vi "Set Setpoint Paramters.vi"(7 "setpoint":string, 8 "error in (no error)":errorcluster, 11 "setpoint cluster":T1={"open-loop controls"={"high pw"=5.0, "low pw"=5.8}, "ramp controls"={"systole"=0.8, "diastole"=0.2}, "blood-pressure controls"={"systole"=0.8, "systole 2"=0.2, "systole 3"=1.0, "systole 4"=0.6}, "sinusoidal controls"={"systole"=0.0, "systole 2"=0.0, "systole 3"=0.0}}) -> (0 "error out":errorcluster, 3 "IA test param out":refnum<class "IA Test Parameters.lvclass">)   [LabVIEW 2020]
uses:
  Parameter Class/IA Test Parameters.lvclass
  Parameter Class/Setpoints/Setpoint Cluster.ctl
  Controls/Open Loop Controls.ctl
  Controls/Ramp Controls.ctl
  Controls/Blood Pressure Controls.ctl
  Controls/sinusoidal controls.ctl
  Parameter Class/Setpoints/Open-loop/Open-Loop Setpoint.lvclass
  C:/Users/jharw/Documents/1 Folder to Rule them All/UMD/Inflation-Apparatus/src/Inflation Test/Parameter Class/IA Test Parameters.lvclass
  Parameter Class/Setpoints/Open-loop/Open-Loop Setpoint.lvclass/Open-Loop Setpoint.ctl
  Parameter Class/Setpoints/Ramp Setpoint/Ramp Setpoint.lvclass
  Parameter Class/Setpoints/Ramp Setpoint/Ramp Setpoint.lvclass/Ramp Setpoint.ctl
  C:/Users/jharw/Documents/1 Folder to Rule them All/UMD/Inflation-Apparatus/src/Inflation Test/Parameter Class/Setpoints/Open-loop/Open-Loop Setpoint.lvclass
  C:/Users/jharw/Documents/1 Folder to Rule them All/UMD/Inflation-Apparatus/src/Inflation Test/Parameter Class/Setpoints/Ramp Setpoint/Ramp Setpoint.lvclass
panel:
  # "SYSTOLE (V):"
  # "DIASTOLE (V):"
  # "FREQUENCY (HZ):"
  # "SYSTOLE (V):"
  # "DIASTOLE (V):"
  # "DICROTIC NOTCH (V):"
  # "FREQUENCY (HZ):"
  # "SYSTOLE (V):"
  # "DIASTOLE (V):"
  # "HIGH PW (%):"
  # "LOW PW (%):"
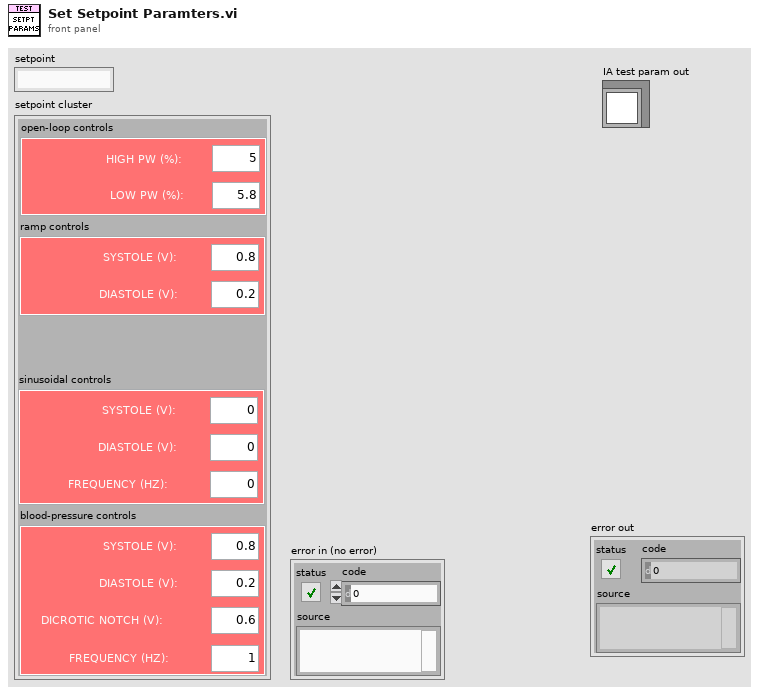
[diagram p1: front panel]
types:
  T1 = typedef "Setpoint Cluster.ctl" = cluster{"open-loop controls":T2, "ramp controls":T3, "blood-pressure controls":T4, "sinusoidal controls":T5}
  T2 = typedef "Open Loop Controls.ctl" = cluster{"high pw":dbl, "low pw":dbl}
  T3 = typedef "Ramp Controls.ctl" = cluster{"systole":dbl, "diastole":dbl}
  T4 = typedef "Blood Pressure Controls.ctl" = cluster{"systole":dbl, "systole 2":dbl, "systole 3":dbl, "systole 4":dbl}
  T5 = typedef "sinusoidal controls.ctl" = cluster{"systole":dbl, "systole 2":dbl, "systole 3":dbl}
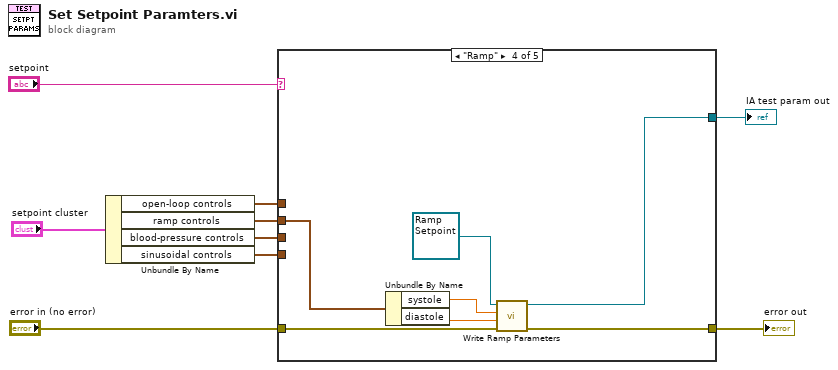
[diagram p0: block diagram]
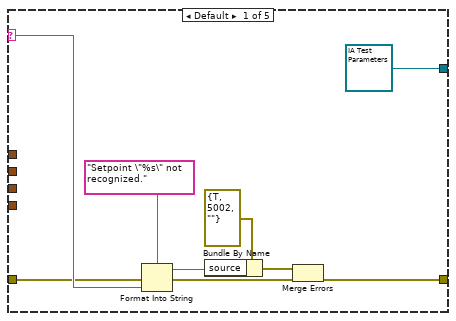
[diagram p2: hidden frame]
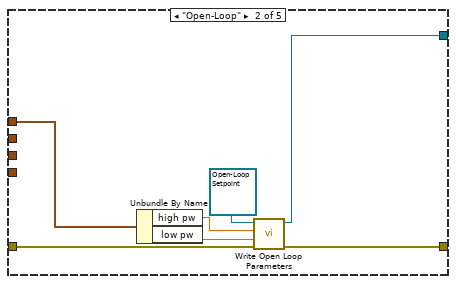
[diagram p3: hidden frame]
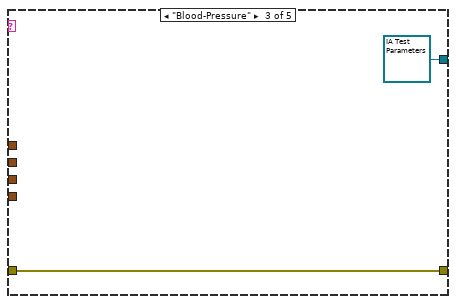
[diagram p4: hidden frame]
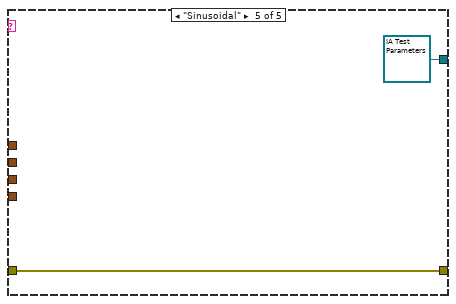
[diagram p5: hidden frame]
diagram:
  n1 = Unbundle By Name("setpoint cluster") -> ("open-loop controls"=w4:T2, "ramp controls"=w3:T3, "blood-pressure controls"=w2:T4, "sinusoidal controls"=w1:T5)
  n2 = case shown="\"Ramp\"" "setpoint" {
    selector: "setpoint" -> [w13 _ _ _ _]
    tunnel: [refnum<class "IA Test Parameters.lvclass"> refnum ("IA Test Parameters.lvclass") w22 refnum<class "IA Test Parameters.lvclass"> refnum ("IA Test Parameters.lvclass") w29 refnum<class "IA Test Parameters.lvclass"> refnum ("IA Test Parameters.lvclass")] -> w6
    tunnel: "error in (no error)" -> [w11 w25 w27 w33 w35]
    tunnel: [w12 w24 w27 w32 w35] -> w9
    tunnel: w4 -> [_ w19 _ _ _]
    tunnel: w3 -> [_ _ _ w28 _]
    tunnel: w2 -> [_ _ _ _ _]
    tunnel: w1 -> [_ _ _ _ _]
    frame Default {
      n3 = Format Into String(format string="Setpoint \"%s\" not recognized.", error in=w11, w13) -> (resulting string=w17:string, error out=w15:errorcluster)  [unwired: 1 in]
      n4 = Bundle By Name(cluster=errorcluster {"status"=TRUE, "code"=5002, "source"=""} ("error out"), "source"=w17) -> (w14:errorcluster)
      n5 = Merge Errors(w14, w15) -> (w12:errorcluster)
    }
    frame "Open-Loop" {
      n6 = Unbundle By Name(w19) -> ("high pw"=w20:dbl, "low pw"=w21:dbl)
      n7 = call "Write Open Loop Parameters.vi"("error in (no error)"=w25, "Low PW"=w21, "High-PW"=w20, "Open-Loop Setpoint in"=refnum<class "Open-Loop Setpoint.lvclass"> refnum) -> ("error out"=w24:errorcluster, "Open-Loop Setpoint out"=w22:refnum<class "Open-Loop Setpoint.lvclass">)  [unwired: 6 in]
    }
    frame "Blood-Pressure" {
    }
    frame "Ramp" {
      n8 = Unbundle By Name(w28) -> ("systole"=w30:dbl, "diastole"=w31:dbl)
      n9 = call "Write Ramp Parameters.vi"("error in (no error)"=w33, "diastole"=w31, "systole"=w30, "Ramp Setpoint in"=refnum<class "Ramp Setpoint.lvclass"> refnum ("Ramp Setpoint.lvclass")) -> ("error out"=w32:errorcluster, "Ramp Setpoint out"=w29:refnum<class "Ramp Setpoint.lvclass">)  [unwired: 6 in]
    }
    frame "Sinusoidal" {
    }
  }
  "error out" <- w9
  "IA test param out" <- w6
